vi "Process.vi"(8 "error in (no error)":errorcluster, 10 "Wash Exit State in":refnum<class "Wash Exit State.lvclass">, 11 "Architecture.lvlib:Thread.lvclass":refnum<class "Thread.lvclass">) -> (0 "error out":errorcluster, 1 "Stop?":bool, 3 "Architecture.lvlib:Thread.lvclass 2":refnum<class "Thread.lvclass">)   [LabVIEW 2019, in "Car Wash Controller.lvlib" / "Wash Exit State.lvclass"]
uses:
  Wash Exit State.lvclass
  Message/Message.lvclass
  Thread/Thread.lvclass
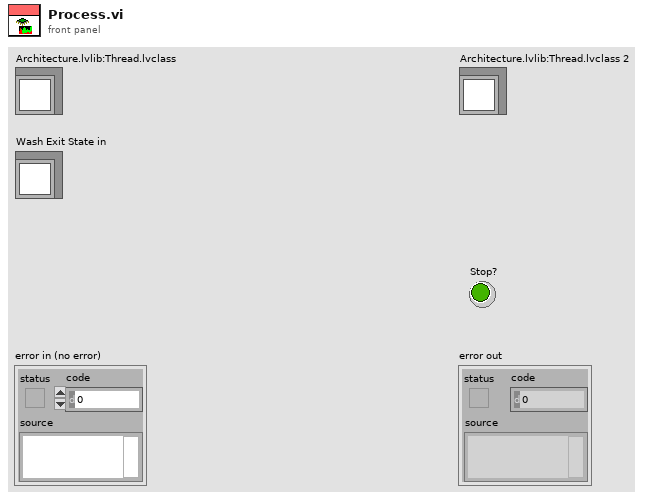
[diagram p1: front panel]
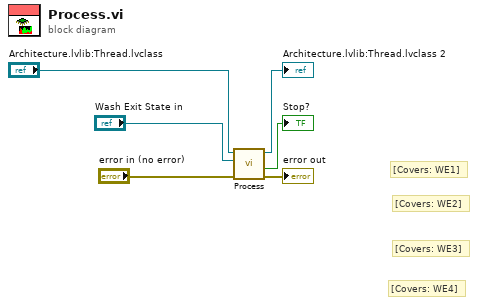
[diagram p0: block diagram]
diagram:
  # "[Covers: WE4]"
  # "[Covers: WE3]"
  # "[Covers: WE2]"
  # "[Covers: WE1]"
  n1 = call-parent "Process.vi"("error in (no error)"="error in (no error)", "Message in"="Wash Exit State in", "Architecture.lvlib:Thread.lvclass"="Architecture.lvlib:Thread.lvclass") -> ("error out"=→"error out":errorcluster, "Stop?"=→"Stop?":bool, "Architecture.lvlib:Thread.lvclass 2"=→"Architecture.lvlib:Thread.lvclass 2":refnum<class "Thread.lvclass">)  [unwired: 6 in]
